vi "GeneratedGetUID.vi"(0 "Text in":refnum<vi>) -> (1 "UID":i32)   [LabVIEW 2013]
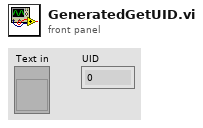
[diagram p1: front panel]
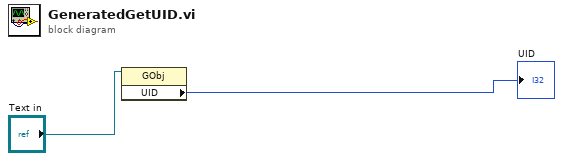
[diagram p0: block diagram]
diagram:
  n1 = property class="GObj"(reference="Text in") -> ("UID"=→"UID":i32)  [unwired: 1 in, 2 out]
